vi "Template.vi"() -> ()   [LabVIEW 2016]
uses:
  <vilib>/NXT/Subs/LVHSConnector.ctl
  <vilib>/NXT/LegoClasses/BrickReference/BrickReference.lvclass
  <vilib>/NXT/Block Support/NXT_InputPort.ctl
  <vilib>/NXT/Block Support/NXT_OutputPort.ctl
  <vilib>/NXT/Dual Mode Library/Sensors/Touch_Pressed.vi
  <vilib>/NXT/Dual Mode Library/Advanced/NXTFlag_Assign.vi
  <vilib>/NXT/Dual Mode Library/Sensors/EV3_Ultrasonic_CM.vi
  <vilib>/NXT/Dual Mode Library/Sensors/readNXTButton.vi
  <vilib>/NXT/Dual Mode Library/Sensors/EV3_Color_Reflect.vi
  <vilib>/NXT/Dual Mode Library/Advanced/NXTFlag_CheckAll.vi
  <vilib>/NXT/NXTIO Xnodes/NXTIONodeSubVIs/NXTMoveMotors.vi
  <vilib>/NXT/NXTIO Xnodes/NXTIOXNode/NXTIO.xnode
panel:
  in  "Color Value":sgl=25.0
  in  "Distance Value":sgl=7.0
  in  "Front Color Port":T1 items=["Port 1", "Port 2", "Port 3", "Port 4"]
  in  "Bumper Port":T1=2 items=["Port 1", "Port 2", "Port 3", "Port 4"]
  in  "Ultrasonic Port":T1=1 items=["Port 1", "Port 2", "Port 3", "Port 4"]
  in  "Rear Color Port":T1=3 items=["Port 1", "Port 2", "Port 3", "Port 4"]
  in  "Motors":cluster{"Left Wheel":T2, "Right Wheel":T2}={"Left Wheel"=0, "Right Wheel"=3} {"Left Wheel" items=["Port A", "Port B", "Port C", "Port D"]; "Right Wheel" items=["Port A", "Port B", "Port C", "Port D"]}
  in  "Robot Reference":T3
  # "Calibration Values"
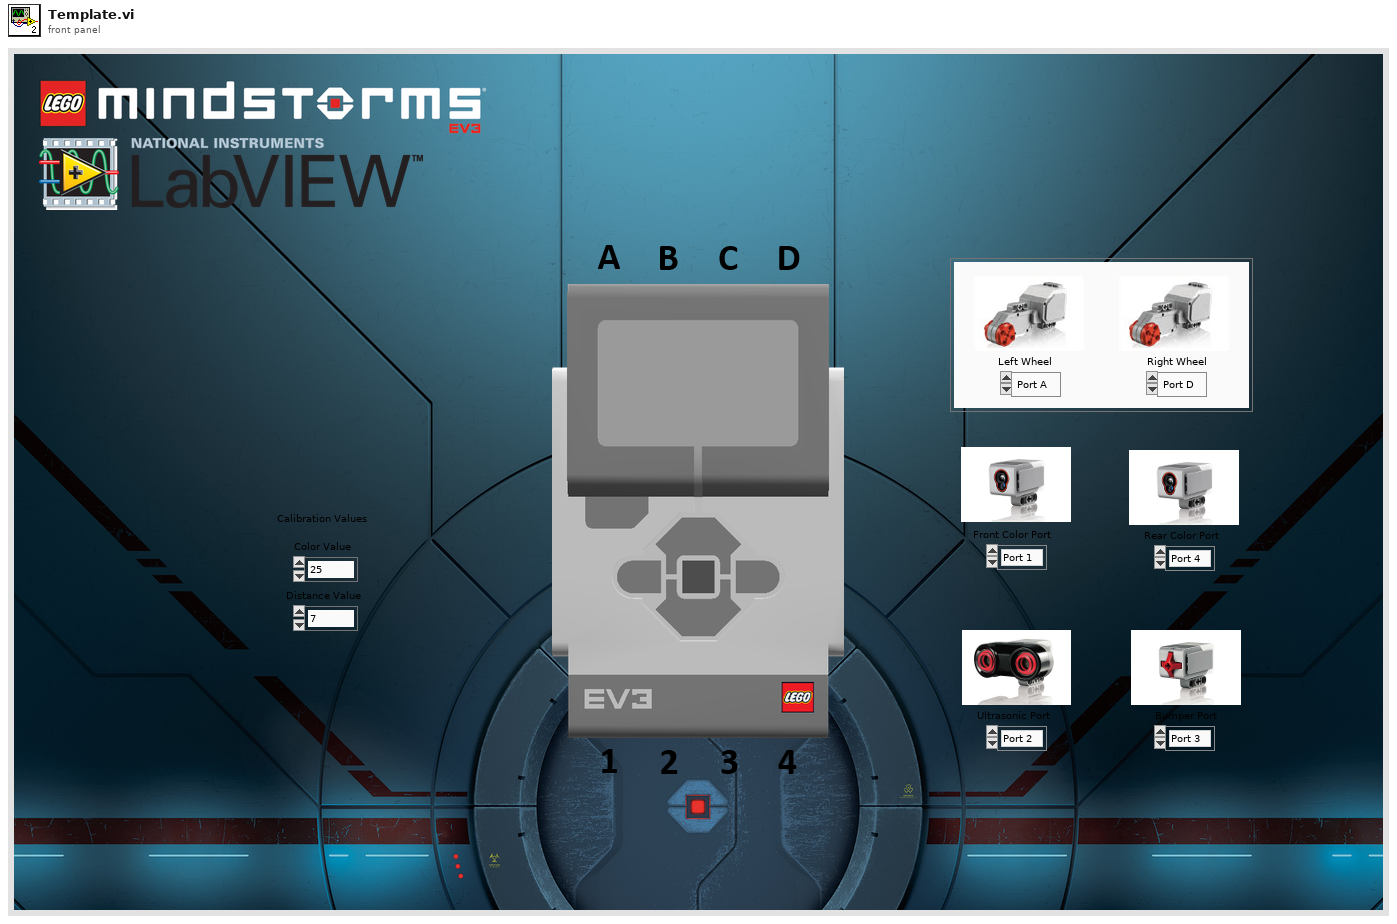
[diagram p1: front panel]
types:
  T1 = typedef "NXT_InputPort.ctl" = u32
  T2 = typedef "NXT_OutputPort.ctl" = u8
  T3 = typedef "LVHSConnector.ctl" = refnum<class "BrickReference.lvclass">
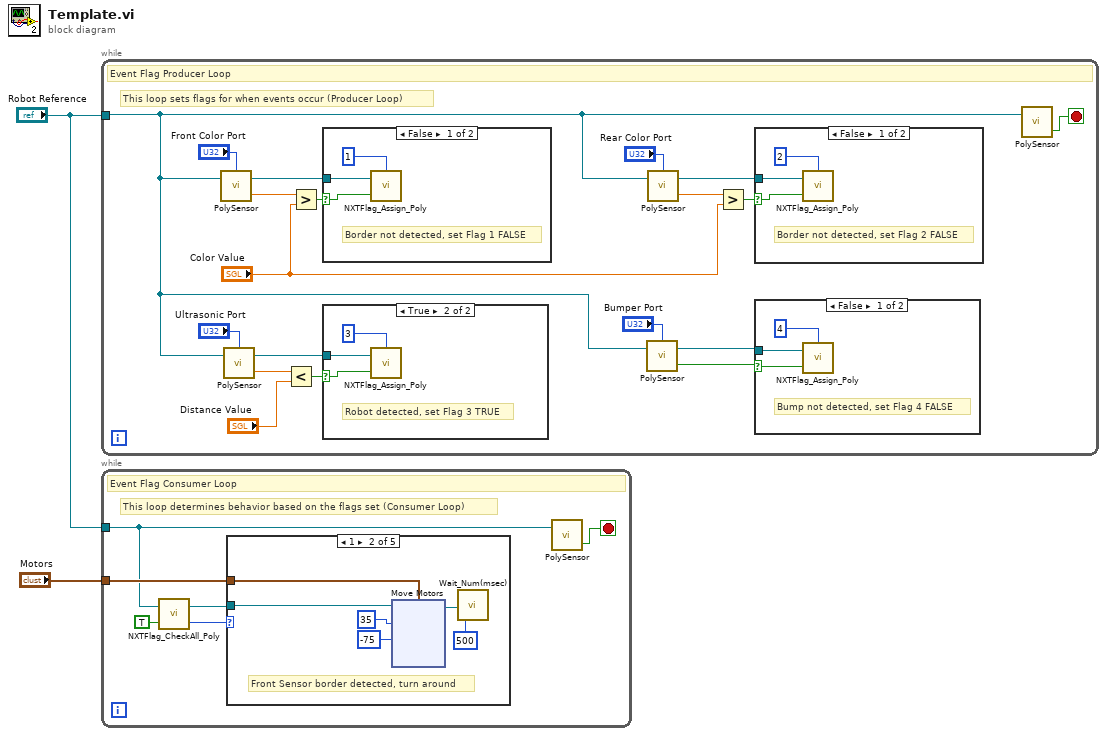
[diagram p0: block diagram]
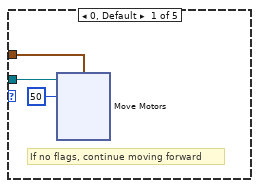
[diagram p2: hidden frame]
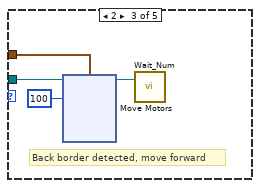
[diagram p3: hidden frame]
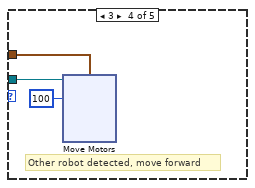
[diagram p4: hidden frame]
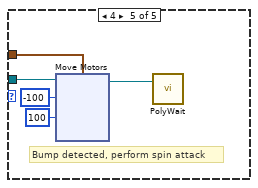
[diagram p5: hidden frame]
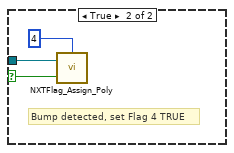
[diagram p6: hidden frame]
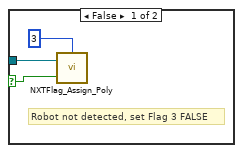
[diagram p7: hidden frame]
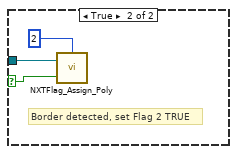
[diagram p8: hidden frame]
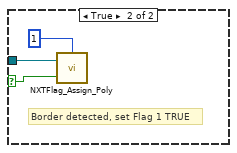
[diagram p9: hidden frame]
diagram:
  n1 = while {
    tunnel: "Robot Reference" -> [w4]
    stop <- w16 stop-if-true
    # "This loop sets flags for when events occur (Producer Loop)"
    # "Event Flag Producer Loop"
    n2 = call-poly <vilib>:"PolySensor.vi"("NXT/EV3"=w4, "Port (Port 1)"="Front Color Port") -> ("Scaled Value"=w21:sgl, "NXT/EV3"=w18:T3)  [unwired: 1 in]
    n3 = call-poly <vilib>:"PolySensor.vi"("NXT/EV3"=w4, "Port (Port 1)"="Ultrasonic Port") -> ("Centimeters"=w11:sgl, "NXT/EV3"=w8:T3)  [unwired: 1 in]
    n4 = Less?(x=w11, y="Distance Value") -> (x < y?=w9:bool)
    n5 = Greater?(x=w21, y="Color Value") -> (0:w19:bool)
    n6 = case shown="False" w19 {
      selector: w19 -> [w41 w43]
      tunnel: w18 -> [w42 w45]
      frame False {
        # "Border not detected, set Flag 1 FALSE"
        n7 = call-poly <vilib>:"NXTFlag_Assign_Poly.vi"("Flag State"=w41, "NXT/EV3"=w42, "NXT/EV3 Flag Number"=i8 1) -> ()  [unwired: 1 in, 1 out]
      }
      frame True {
        # "Border detected, set Flag 1 TRUE"
        n8 = call-poly <vilib>:"NXTFlag_Assign_Poly.vi"("Flag State"=w43, "NXT/EV3"=w45, "NXT/EV3 Flag Number"=i8 1) -> ()  [unwired: 1 in, 1 out]
      }
    }
    n9 = case shown="True" w9 {
      selector: w9 -> [w29 w31]
      tunnel: w8 -> [w30 w33]
      frame False {
        # "Robot not detected, set Flag 3 FALSE"
        n10 = call-poly <vilib>:"NXTFlag_Assign_Poly.vi"("Flag State"=w29, "NXT/EV3"=w30, "NXT/EV3 Flag Number"=i8 3) -> ()  [unwired: 1 in, 1 out]
      }
      frame True {
        # "Robot detected, set Flag 3 TRUE"
        n11 = call-poly <vilib>:"NXTFlag_Assign_Poly.vi"("Flag State"=w31, "NXT/EV3"=w33, "NXT/EV3 Flag Number"=i8 3) -> ()  [unwired: 1 in, 1 out]
      }
    }
    n12 = call-poly <vilib>:"PolySensor.vi"("NXT/EV3"=w4, "Port (Port 1)"="Bumper Port") -> ("Yes / No"=w3:bool, "NXT/EV3"=w6:T3)  [unwired: 1 in]
    n13 = call-poly <vilib>:"PolySensor.vi"("NXT/EV3"=w4, "Port (Port 1)"="Rear Color Port") -> ("Scaled Value"=w20:sgl, "NXT/EV3"=w17:T3)  [unwired: 1 in]
    n14 = Greater?(x=w20, y="Color Value") -> (0:w15:bool)
    n15 = case shown="False" w15 {
      selector: w15 -> [w35 w37]
      tunnel: w17 -> [w36 w39]
      frame False {
        # "Border not detected, set Flag 2 FALSE"
        n16 = call-poly <vilib>:"NXTFlag_Assign_Poly.vi"("Flag State"=w35, "NXT/EV3"=w36, "NXT/EV3 Flag Number"=i8 2) -> ()  [unwired: 1 in, 1 out]
      }
      frame True {
        # "Border detected, set Flag 2 TRUE"
        n17 = call-poly <vilib>:"NXTFlag_Assign_Poly.vi"("Flag State"=w37, "NXT/EV3"=w39, "NXT/EV3 Flag Number"=i8 2) -> ()  [unwired: 1 in, 1 out]
      }
    }
    n18 = case shown="False" w3 {
      selector: w3 -> [w23 w25]
      tunnel: w6 -> [w24 w27]
      frame False {
        # "Bump not detected, set Flag 4 FALSE"
        n19 = call-poly <vilib>:"NXTFlag_Assign_Poly.vi"("Flag State"=w23, "NXT/EV3"=w24, "NXT/EV3 Flag Number"=i8 4) -> ()  [unwired: 1 in, 1 out]
      }
      frame True {
        # "Bump detected, set Flag 4 TRUE"
        n20 = call-poly <vilib>:"NXTFlag_Assign_Poly.vi"("Flag State"=w25, "NXT/EV3"=w27, "NXT/EV3 Flag Number"=i8 4) -> ()  [unwired: 1 in, 1 out]
      }
    }
    n21 = call-poly <vilib>:"PolySensor.vi"("NXT/EV3"=w4) -> ("Yes/No"=w16:bool)  [unwired: 2 in, 1 out]
  }
  n22 = while {
    tunnel: "Robot Reference" -> [w47]
    tunnel: "Motors" -> [w49]
    stop <- w48 stop-if-true
    # "This loop determines behavior based on the flags set (Consumer Loop)"
    # "Event Flag Consumer Loop"
    n23 = call-poly <vilib>:"NXTFlag_CheckAll_Poly.vi"("Clear if Found"=TRUE, "NXT/EV3"=w47) -> ("NXT/EV3 Flag Number"=w51:i32, "NXT/EV3"=w50:T3)  [unwired: 1 in]
    n24 = case shown="1" w51 {
      tunnel: w50 -> [w53 w68 w79 w91 w102]
      tunnel: w49 -> [w54 w67 w80 w90 w104]
      frame 0, Default {
        w52 = i8 50 ("Power/Speed 1")
        # "If no flags, continue moving forward"
        n25 = xnode "Move Motors"("Power/Speed 1"=w52, "Motors"=w54, "NXT/EV3"=w53, "Power/Speed 2"=w52) -> ()  [unwired: 1 out]
      }
      frame 1 {
        # "Front Sensor border detected, turn around"
        n26 = xnode "Move Motors"("Power/Speed 1"=i8 35, "Motors"=w67, "NXT/EV3"=w68, "Power/Speed 2"=i8 -75) -> ("NXT/EV3"=w65:T3)
        n27 = call <vilib>:"Wait_Num(msec).vi"("Time (100 msec)"=u32 500, "NXT/EV3"=w65) -> ()  [unwired: 2 in, 1 out]
      }
      frame 2 {
        # "Back border detected, move forward"
        n28 = xnode "Move Motors"("Power/Speed 1"=i8 100, "Motors"=w80, "NXT/EV3"=w79) -> ("NXT/EV3"=w77:T3)  [unwired: 1 in]
        n29 = call <vilib>:"Wait_Num.vi"("NXT/EV3"=w77) -> ()  [unwired: 3 in, 1 out]
      }
      frame 3 {
        # "Other robot detected, move forward"
        n30 = xnode "Move Motors"("Power/Speed 1"=i8 100, "Motors"=w90, "NXT/EV3"=w91) -> ()  [unwired: 1 in, 1 out]
      }
      frame 4 {
        # "Bump detected, perform spin attack"
        n31 = xnode "Move Motors"("Power/Speed 1"=i8 -100, "Motors"=w104, "NXT/EV3"=w102, "Power/Speed 2"=i8 100) -> ("NXT/EV3"=w103:T3)
        n32 = call-poly <vilib>:"PolyWait.vi"("NXT/EV3"=w103) -> ()  [unwired: 3 in, 1 out]
      }
    }
    n33 = call-poly <vilib>:"PolySensor.vi"("NXT/EV3"=w47) -> ("Yes/No"=w48:bool)  [unwired: 2 in, 1 out]
  }
